vi "Merge_Errors.vi"(8 "Error 2":errorcluster, 11 "Error 1":errorcluster) -> (0 "Error Out":errorcluster)   [LabVIEW 2012, in "AccelNET.lvlib" / "Useful_SubVIs.lvlib"]
uses:
  Useful_SubVIs.lvlib
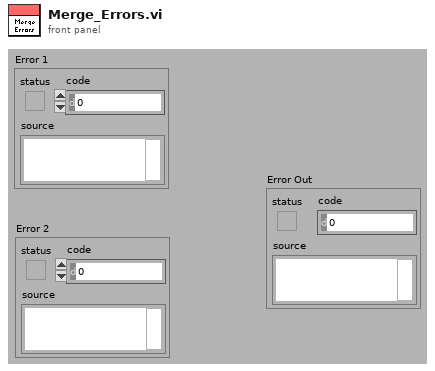
[diagram p1: front panel]
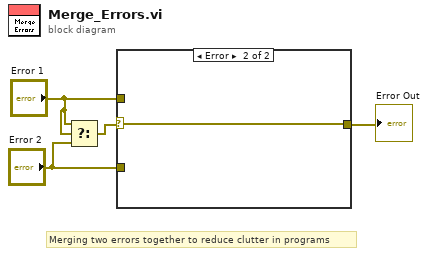
[diagram p0: block diagram]
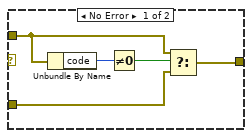
[diagram p2: hidden frame]
diagram:
  # "Merging two errors together to reduce clutter in programs"
  n1 = Select(t="Error 1", s="Error 1", f="Error 2") -> (s? t:f=w4:errorcluster)
  n2 = case shown="Error" w4 {
    selector: w4 -> [_ w10]
    tunnel: "Error 1" -> [w5 _]
    tunnel: "Error 2" -> [w7 _]
    tunnel: [w6 w10] -> w1
    frame No Error {
      n3 = Unbundle By Name(w5) -> ("code"=w9:i32)
      n4 = Not Equal To 0?(x=w9) -> (x != 0?=w8:bool)
      n5 = Select(t=w5, s=w8, f=w7) -> (s? t:f=w6:errorcluster)
    }
    frame Error {
    }
  }
  "Error Out" <- w1
